vi "NetVarWrite_dbl.vi"(8 "error in (no error)":errorcluster, 10 "Numeric":dbl, 11 "Refnum in":refnum<k21>) -> (0 "error out":errorcluster)   [LabVIEW 2013]
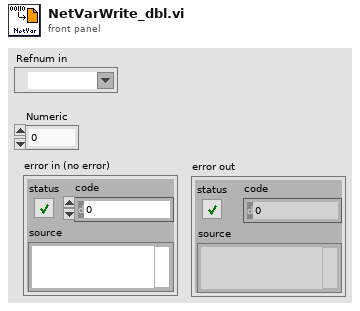
[diagram p1: front panel]
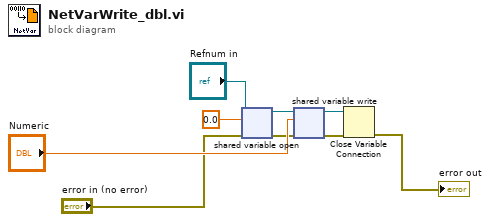
[diagram p0: block diagram]
diagram:
  n1 = shared-variable-open("Refnum in", "error in (no error)", 0.0) -> (w5:refnum<k21>, w4:errorcluster)  [unwired: 1 in]
  n2 = shared-variable-write(w5, w4, "Numeric") -> (w6:refnum<k21>, w3:errorcluster)
  n3 = Close Variable Connection(8:w3, 11:w6) -> (0:→"error out":errorcluster)
